vi "Spline Interpolation PtByPt.vi"(2 "sample length":i32=100, 3 "initialize":bool, 4 "Interpolant":dbl[](array[numeric]), 5 "x value":dbl format="%0.2f", 6 "x":dbl format="%0.2f", 7 "y":dbl format="%0.2f") -> (0 "error":i32, 1 "interpolation value":dbl format="%0.2f")   [LabVIEW 2020, in "NI_PtbyPt.lvlib"]
doc: "Performs a cubic spline interpolation of f at <B>x</B>, given a set of tabulated values."
uses:
  NI_PtbyPt.lvlib
  NI_AALPro.lvlib
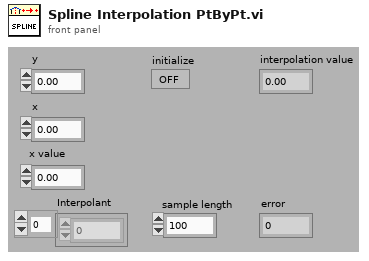
[diagram p1: front panel]
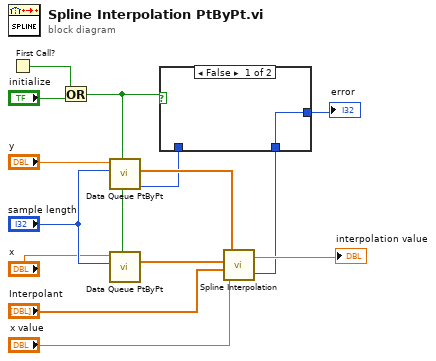
[diagram p0: block diagram]
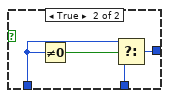
[diagram p2: hidden frame]
diagram:
  n1 = First Call?() -> (First Call?: T/F=w1:bool)
  n2 = Or(x=w1, y="initialize") -> (x .or. y?=w2:bool)
  n3 = call "Data Queue PtByPt.vi"("initialize"=w2, "sample length"="sample length", "input data point"="y") -> ("error"=w6:i32, "Current Queue"=w11:dbl[])  [unwired: 4 in, 3 out]
  n4 = call "Data Queue PtByPt.vi"("initialize"=w2, "sample length"="sample length", "input data point"="x") -> ("Current Queue"=w10:dbl[])  [unwired: 4 in, 4 out]
  n5 = call "Spline Interpolation.vi"("x value"="x value", "Interpolant"="Interpolant", "X"=w10, "Y"=w11) -> ("error"=w4:i32, "interpolation value"=→"interpolation value":dbl)
  n6 = case shown="False" w2 {
    tunnel: w6 -> [_ w18]
    tunnel: w4 -> [w15 w17]
    tunnel: [w15 w16] -> w5
    frame False {
    }
    frame True {
      n7 = Not Equal To 0?(x=w18) -> (x != 0?=w19:bool)
      n8 = Select(t=w18, s=w19, f=w17) -> (s? t:f=w16:i32)
    }
  }
  "error" <- w5
